vi "DAQ_DIS.vi"(6 "Slot":T1, 8 "error in":errorcluster, 11 "CHS":string[](array[string])=["PASSButton", "FAILButton"]) -> (0 "error out":errorcluster, 3 "data":bool[](array[boolean]))   [LabVIEW 2013]
uses:
  SystemCode/SysControl/Slot.ctl
  <vilib>/DAQmx/read.llb/DAQmx Read (Digital 1D Bool NChan 1Samp 1Line).vi
  SourceCode/GlobalValue.vi
  <vilib>/DAQmx/create/channels.llb/DAQmx Create Channel (DI-Digital Input).vi
  <vilib>/Utility/error.llb/Error Cluster From Error Code.vi
  <vilib>/DAQmx/miscellaneous.llb/DAQmx Fill In Error Info.vi
  <vilib>/ErrorRing/Error Ring.xnode
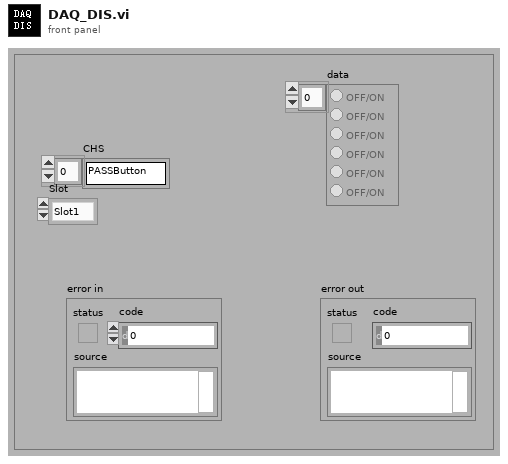
[diagram p1: front panel]
types:
  T1 = typedef "Slot.ctl" = enum16{"Slot1", "Slot2", "Slot3", "Slot4"}
  T2 = typedef "DAQConfig.ctl" = cluster{"DIO":string[][], "AO":string[][], "AI":string[][]}
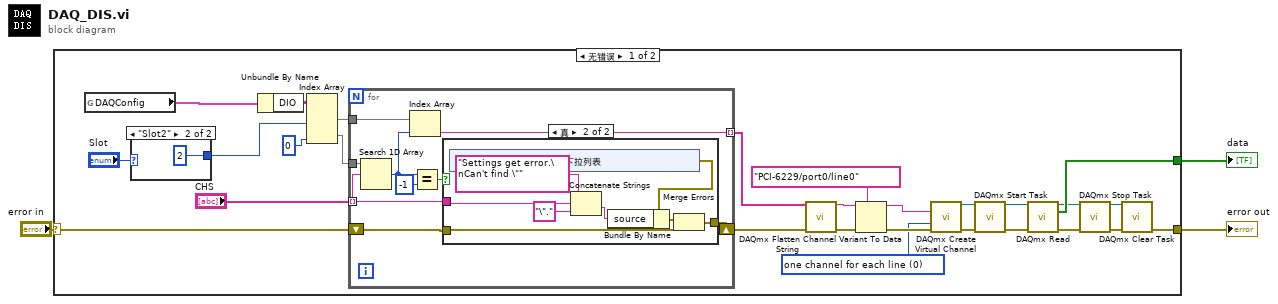
[diagram p0: block diagram]
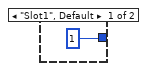
[diagram p2: hidden frame]
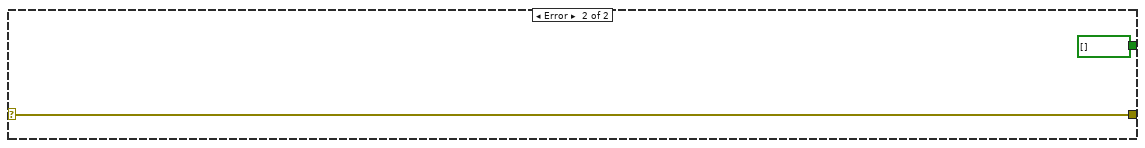
[diagram p4: hidden frame]
diagram:
  n1 = case shown="无错误" "error in" {
    selector: "error in" -> [w10 w56]
    tunnel: [w30 w56] -> w3
    tunnel: [w29 bool[] [] ("data")] -> w2
    frame No Error {
      w15 = 0 items=["one channel for each line", "one channel for all lines"] ("line grouping")
      n2 = global read "GlobalValue.vi" "DAQConfig"() -> (w4:T2)
      n3 = case shown="\"Slot2\"" "Slot" {
        tunnel: [1 ("索引 (行)") 2 ("索引 (行)")] -> w6
        frame "Slot1", Default {
        }
        frame "Slot2" {
        }
      }
      n4 = Unbundle By Name(w4) -> ("DIO"=w13:string[][])
      n5 = Index Array(array=w13, index (col) #1=w6, index (col) #2=0 ("索引 (列)")) -> (element #1=w11:string[], element #2=w12:string[])  [unwired: 2 in]
      n6 = for {
        tunnel: "CHS" -> [w41] mode=indexing
        tunnel: w12 -> [w37]
        tunnel: w11 -> [w36]
        shift-right: [w34] -> w9
        shift-left: w10 -> [w35]
        tunnel: [w33] -> w7 mode=indexing
        n7 = Search 1D Array(1D array=w37, element=w41) -> (index of element=w38:i32)  [unwired: 1 in]
        n8 = Index Array(array=w36, index=w38) -> (element=w33:string)
        n9 = Equal?(x=w38, y=-1) -> (x = y?=w40:bool)
        n10 = case shown="真" w40 {
          tunnel: w41 -> [_ w46]
          tunnel: w35 -> [w42 w45]
          tunnel: [w42 w44] -> w34
          frame False {
          }
          frame True {
            n11 = xnode "错误下拉列表"() -> ("错误输出"=w43:errorcluster)
            n12 = Concatenate Strings("Settings get error.\nCan't find \"" ("message"), w46, "\"." ("string")) -> (w49:string)
            n13 = Bundle By Name(cluster=w43, "source"=w49) -> (w48:errorcluster)
            n14 = Merge Errors(w48, w45) -> (w44:errorcluster)
          }
        }
      }
      n15 = call <vilib>:"DAQmx Flatten Channel String.vi"("names in"=w7, "error in"=w9) -> ("names out"=w21:string, "error out"=w19:errorcluster)  [unwired: 12 in]
      n16 = Variant To Data(error in=w19, type=tag "PCI-6229/port0/line0" ("lines"), Variant=w21) -> (data=w20:tag, error out=w18:errorcluster)
      n17 = call-poly <vilib>:"DAQmx Create Virtual Channel.vi"("lines"=w20, "line grouping"=w15, "error in"=w18) -> ("task out"=w28:refnum<k21>, "error out"=w27:errorcluster)  [unwired: 11 in]
      n18 = call <vilib>:"DAQmx Start Task.vi"("task/channels in"=w28, "error in"=w27) -> ("task out"=w26:refnum<k21>, "error out"=w25:errorcluster)  [unwired: 12 in]
      n19 = call-poly <vilib>:"DAQmx Read.vi"("task/channels in"=w26, "error in"=w25) -> ("task out"=w17:refnum<k21>, "data"=w29:bool[], "error out"=w16:errorcluster)  [unwired: 11 in]
      n20 = call <vilib>:"DAQmx Stop Task.vi"("task/channels in"=w17, "error in"=w16) -> ("task out"=w24:refnum<k21>, "error out"=w23:errorcluster)  [unwired: 12 in]
      n21 = call <vilib>:"DAQmx Clear Task.vi"("task in"=w24, "error in"=w23) -> ("error out"=w30:errorcluster)  [unwired: 13 in]
    }
    frame Error {
    }
  }
  "error out" <- w3
  "data" <- w2
